vi "MDAQ_RawDataParser.vi"(8 "error in":errorcluster, 11 "Raw Data In":string[](array[string])) -> (0 "error out":errorcluster, 2 "Run Data Cluster":T1 {"Temperature B" scale=0.0..100.0; "Temperature A" scale=0.0..100.0})   [LabVIEW 2021]
uses:
  DAT_Cluster.ctl
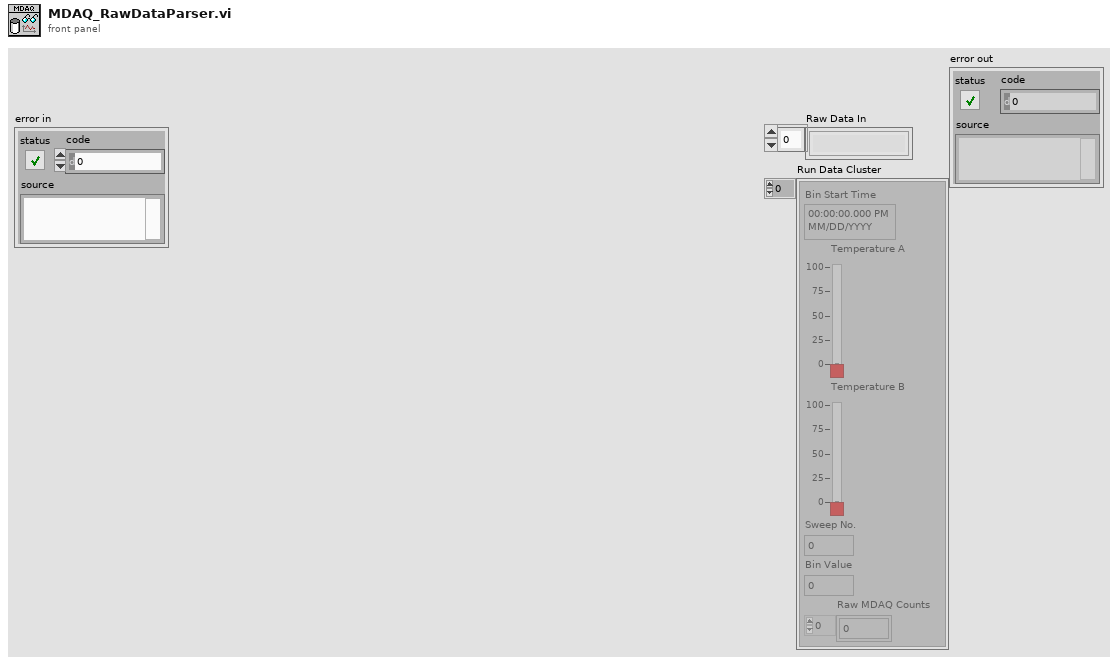
[diagram p1: front panel]
types:
  T1 = typedef "DAT_Cluster.ctl" = cluster{"Bin Start Time":timestamp, "Temperature A":dbl, "Temperature B":dbl, "Sweep No.":i32, "Bin Value":i32, "Raw MDAQ Counts":i32[]}[]
  T2 = cluster{"Bin Start Time":timestamp, "Temperature A":dbl, "Temperature B":dbl, "Sweep No.":i32, "Bin Value":i32, "Raw MDAQ Counts":i32[]}
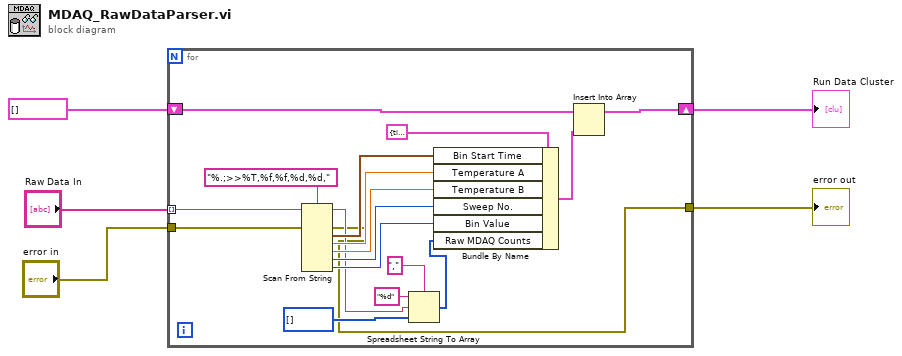
[diagram p0: block diagram]
diagram:
  n1 = for {
    tunnel: "Raw Data In" -> [w23] mode=indexing
    tunnel: "error in" -> [w22]
    shift-right: [w12] -> w2
    shift-left: T1 [] ("Run Data Cluster") -> [w20]
    tunnel: [w6] -> w1
    n2 = Scan From String(format string="%.;>>%T,%f,%f,%d,%d,", input string=w23, error in=w22) -> (remaining string=w10:string, error out=w6:errorcluster, output 1=w17:timestamp, output 2=w16:dbl, output 3=w15:dbl, output 4=w14:i32, output 5=w13:i32)  [unwired: 6 in, 1 out]
    n3 = Spreadsheet String To Array(delimiter (Tab)=",", format string="%d", spreadsheet string=w10, array type (2D Dbl)=i32[] [] ("Raw MDAQ Counts")) -> (array=w8:i32[])
    n4 = Bundle By Name(cluster=T2 {"Bin Start Time"=timestamp(0 s since 1904-01-01), "Temperature A"=0.0, "Temperature B"=0.0, "Sweep No."=0, "Bin Value"=0, "Raw MDAQ Counts"=[]} ("new element/subarray"), "Bin Start Time"=w17, "Temperature A"=w16, "Temperature B"=w15, "Sweep No."=w14, "Bin Value"=w13, "Raw MDAQ Counts"=w8) -> (w18:T2)
    n5 = Insert Into Array(array=w20, new element=w18) -> (w12:T1)  [unwired: 1 in]
  }
  "Run Data Cluster" <- w2
  "error out" <- w1
